vi "Self Test.vi"(8 "error in":errorcluster, 11 "69X_79X in":refnum<class "69X_79X.lvclass">) -> (0 "error out":errorcluster, 3 "69X_79X out":refnum<class "69X_79X.lvclass">)   [LabVIEW 2019, in "69X_79X.lvlib" / "69X_79X.lvclass"]
uses:
  Library/69X_79X.lvclass
  Library/69X_79X.lvclass/69X_79X.ctl
  builds/Instruments/PowerSupply.lvlibp/Library/PowerSupply.lvclass
  <instrlib>/Agilent N6900 N7900 Series/Agilent N6900 N7900 Series.lvlib
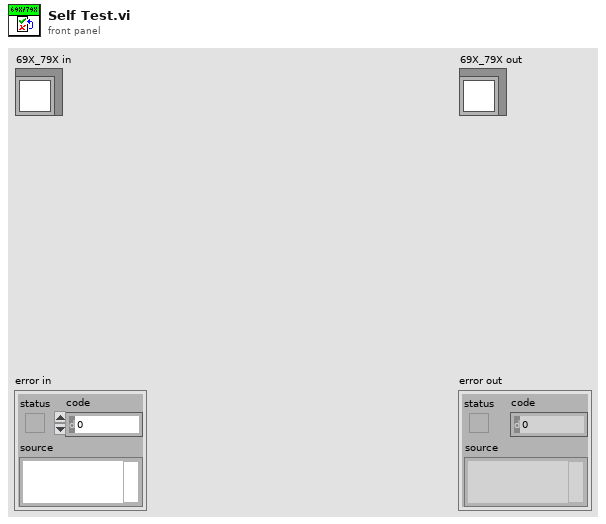
[diagram p1: front panel]
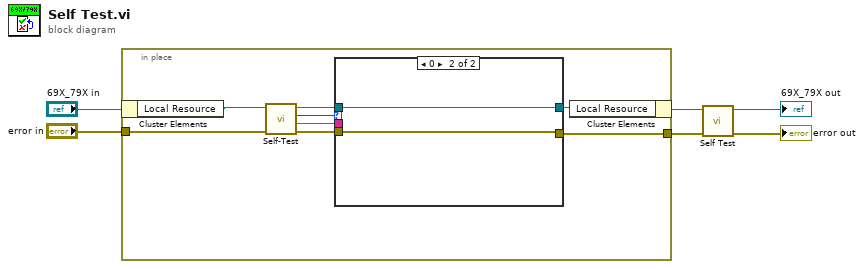
[diagram p0: block diagram]
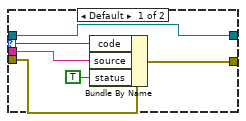
[diagram p2: hidden frame]
diagram:
  n1 = in-place {
    in-place-border: "error in" -> [w13]
    in-place-border: [w7] -> w2
    n2 = in-place-cluster #1("69X_79X in") -> ("Local Resource"=w14:refnum<visa-resource-name>)
    n3 = call <instrlib>:"Self-Test.vi"("error in (no error)"=w13, "VISA resource name"=w14) -> ("error out"=w10:errorcluster, "Self-Test Result Message"=w9:string, "Self-Test Result Code"=w12:i32, "VISA resource name out"=w11:refnum<visa-resource-name>)  [unwired: 6 in]
    n4 = case shown="0" w12 {
      selector: w12 -> [w19 _]
      tunnel: w11 -> [w15 w21]
      tunnel: w10 -> [w20 w22]
      tunnel: w9 -> [w18 _]
      tunnel: [w16 w22] -> w7
      tunnel: [w15 w21] -> w8
      frame Default {
        n5 = Bundle By Name(cluster=w20, "code"=w19, "source"=w18, "status"=TRUE) -> (w16:errorcluster)
      }
      frame 0 {
      }
    }
    n6 = in-place-cluster #1("Local Resource"=w8) -> (w4:refnum<class "69X_79X.lvclass">)
  }
  n7 = call-parent "Self Test.vi"("error in"=w2, "Instruments in"=w4) -> ("error out"=→"error out":errorcluster, "Instruments out"=→"69X_79X out":refnum<class "69X_79X.lvclass">)  [unwired: 8 in]
